vi "UART_readline.vi"(8 "error in (no error)":errorcluster, 11 "VISA Refnum in":refnum<visa-resource-name>) -> (0 "error out":errorcluster, 2 "Input string":string, 3 "VISA Refnum out":refnum<visa-resource-name>)   [LabVIEW 2017]
panel:
  out "input buffer":string
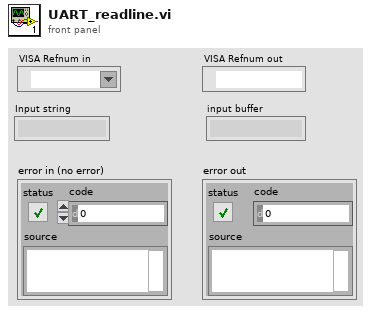
[diagram p1: front panel]
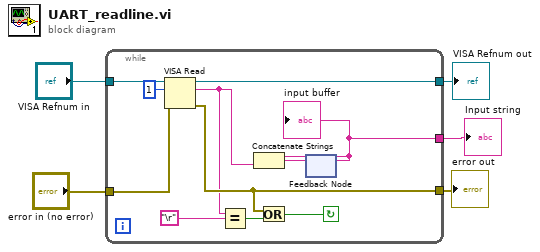
[diagram p0: block diagram]
diagram:
  n1 = while {
    tunnel: [w16] -> w2
    tunnel: "error in (no error)" -> [w15]
    tunnel: [w12] -> w3
    tunnel: "VISA Refnum in" -> [w10]
    tunnel: [w6] -> w1
    stop <- w14 continue-if-true
    n2 = VISA Read(VISA resource name=w10, byte count=u32 1, error in (no error)=w15) -> (VISA resource name out=w16:refnum<visa-resource-name>, read buffer=w7:string, error out=w12:errorcluster)  [unwired: 1 out]
    n3 = Equal?(x=w7, y="\r") -> (x = y?=w13:bool)
    n4 = Or(x=w12, y=w13) -> (x .or. y?=w14:bool)
    n5 = feedback #1() -> (w6:string)  [unwired: 1 in]
    "input buffer" <- w6
    n6 = Concatenate Strings(w6, w7) -> (w8:string)
    n7 = feedback-in #1(w8) -> ()
  }
  "error out" <- w3
  "VISA Refnum out" <- w2
  "Input string" <- w1
